vi "sum.vi"(2 "+1":bool, 3 "B":T1, 4 "A":T3) -> (0 "C":bool, 1 "Output":T2)   [LabVIEW 2013]
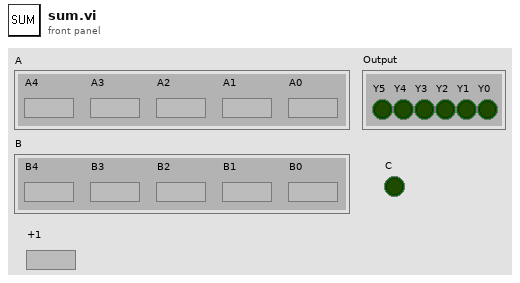
[diagram p1: front panel]
types:
  T1 = cluster{"B4":bool, "B3":bool, "B2":bool, "B1":bool, "B0":bool}
  T2 = cluster{"Y5":bool, "Y4":bool, "Y3":bool, "Y2":bool, "Y1":bool, "Y0":bool}
  T3 = cluster{"A4":bool, "A3":bool, "A2":bool, "A1":bool, "A0":bool}
  T4 = cluster{"C":bool, "S":bool, "S":bool, "S":bool, "S":bool, "S":bool}
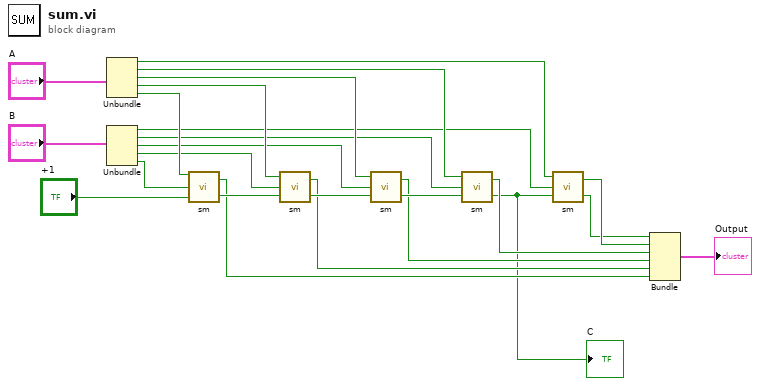
[diagram p0: block diagram]
diagram:
  n1 = Unbundle("A") -> ("A4"=w14:bool, "A3"=w15:bool, "A2"=w16:bool, "A1"=w17:bool, "A0"=w19:bool)
  n2 = Unbundle("B") -> ("B4"=w10:bool, "B3"=w11:bool, "B2"=w12:bool, "B1"=w13:bool, "B0"=w18:bool)
  n3 = call "sm.vi"("c"="+1", "b"=w18, "a"=w19) -> ("C"=w20:bool, "S"=w9:bool)
  n4 = call "sm.vi"("c"=w20, "b"=w13, "a"=w17) -> ("C"=w21:bool, "S"=w8:bool)
  n5 = call "sm.vi"("c"=w21, "b"=w12, "a"=w16) -> ("C"=w22:bool, "S"=w7:bool)
  n6 = call "sm.vi"("c"=w22, "b"=w11, "a"=w15) -> ("C"=w1:bool, "S"=w6:bool)
  "C" <- w1
  n7 = call "sm.vi"("c"=w1, "b"=w10, "a"=w14) -> ("C"=w4:bool, "S"=w5:bool)
  n8 = Bundle("C"=w4, "S"=w5, "S"=w6, "S"=w7, "S"=w8, "S"=w9) -> (→"Output":T4)  [unwired: 1 in]
